vi "CRYGet Channel Name Dialog.vi"(10 "Channel Name":string caption="µÑ\\¸tÇ„¹DÇ …Ç%¸XÕíÂÜÂ$Æ.", 11 "Window Title":string) -> (2 "Channel Name Out":string, 3 "Return Flag":bool)   [LabVIEW 2013]
panel:
  in  "Cancel":bool
  in  "OK":bool
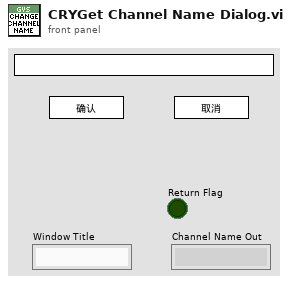
[diagram p1: front panel]
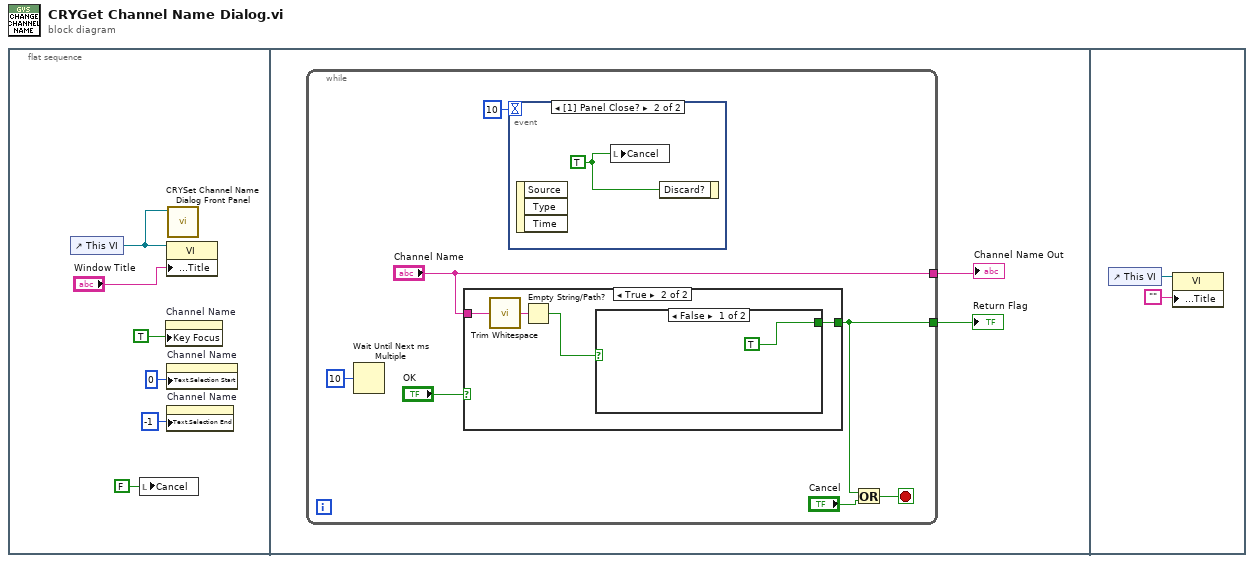
[diagram p0: block diagram]
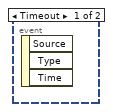
[diagram p2: hidden frame]
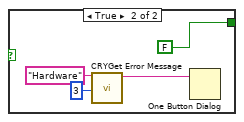
[diagram p4: hidden frame]
diagram:
  n1 = flat-sequence {
    frame #0 {
      n2 = control-ref of="This VI"() -> (w2:refnum<vi>)
      n3 = local write "Cancel"(FALSE ("Cancel")) -> ()
      n4 = property on="Channel Name" class="Str"("Key Focus"=TRUE) -> ()  [unwired: 2 in, 2 out]
      n5 = property class="VI"(reference=w2, "Front Panel.Title"="Window Title") -> ()  [unwired: 1 in, 2 out]
      n6 = property on="Channel Name" class="Str"("Text.Selection Start"=u32 0 ("Text.Selection:Start")) -> ()  [unwired: 2 in, 2 out]
      n7 = property on="Channel Name" class="Str"("Text.Selection End"=-1 ("Text.Selection:End")) -> ()  [unwired: 2 in, 2 out]
      n8 = call "CRYSet Channel Name Dialog Front Panel.vi"("Vi Ref"=w2) -> ()  [unwired: 11 in]
    }
    frame #1 {
      n9 = while {
        tunnel: ["Channel Name"] -> w8
        tunnel: [w10] -> w7
        stop <- w15 stop-if-true
        n10 = Wait Until Next ms Multiple(millisecond multiple=u32 10) -> ()  [unwired: 1 out]
        n11 = case shown="True" "OK" {
          selector: "OK" -> [w17 _]
          tunnel: [w17 w19] -> w10
          tunnel: "Channel Name" -> [_ w21]
          frame False {
          }
          frame True {
            n12 = call <vilib>:"Trim Whitespace.vi"("string"=w21) -> ("trimmed string"=w18:string)  [unwired: 1 in]
            n13 = Empty String/Path?(string/path=w18) -> (empty?=w20:bool)
            n14 = case shown="False" w20 {
              tunnel: [TRUE ("empty?") FALSE ("empty?")] -> w19
              frame False {
              }
              frame True {
                n15 = call "CRYGet Error Message.vi"("Error No"=3 ("No"), "Kind"="Hardware") -> ("Message"=w23:string)  [unwired: 4 in, 5 out]
                n16 = One Button Dialog(message=w23) -> ()  [unwired: 2 out]
              }
            }
          }
        }
        n17 = event shown="[1] Panel Close?" {
          selector: _ -> [_ _]
          dyn-events: _ -> [_ _]
          timeout: 10 -> [_ _]
          event Timeout {
            n18 = event-data() -> ()  [unwired: 1 in, 3 out]
          }
          event Panel Close? {
            w16 = TRUE ("OK")
            n19 = event-data() -> ()  [unwired: 1 in, 3 out]
            n20 = local write "Cancel"(w16) -> ()
            n21 = event-data("Discard?"=w16) -> ()  [unwired: 1 in, 1 out]
          }
        }
        n22 = Or(x=w10, y="Cancel") -> (x .or. y?=w15:bool)
      }
      "Return Flag" <- w7
      "Channel Name Out" <- w8
    }
    frame #2 {
      n23 = control-ref of="This VI"() -> (w28:refnum<vi>)
      n24 = property class="VI"(reference=w28, "Front Panel.Title"="") -> ()  [unwired: 1 in, 2 out]
    }
  }
